vi "ValveFSM.vi"(7 "ReadOnlyIn":T4={"Qref"={"ValveCTR"=refnum, "Error"=refnum}, "UI_EN"=FALSE, "UserEventREF"={"TimeBasedProducer"={"Reg"=refnum, "Ref"=refnum}, "TimeBasedTempRead"={"Reg"=refnum, "Ref"=refnum}}, "UI_REF"=variant, "Paths"={"Log_Dir"=path "", "TempLog"=path "", "WateringLog"=path "", "Error"=path "", "Settings_Dir"=path "", "CFG.ini"=path "", "Plant_Digital_OP"=path "", "TimeTable"=path "", "Consol_Dir"=path "", "Input"=path "", "Output"=path "", "Timeout"=path "", "TimeoutTable"=path "", "Ch_Stat"=path "", "Temp"=path ""}, "PI_REF"={"IO"=enum."Remote", "Interface"=enum."Serial", "LINX Device Config"={"Interface"=enum."Serial", "COM Port"="", "TCP Configuration"={"IP Address"="", "Port"=0}, "Device Family"=0, "Device ID"=0, "Device Name"="", "TCP Ref"=refnum, "Channels"={"DI"=[], "DO"=[], "AI"=[], "AO"=[], "PWM"=[], "QE"=[], "UART"=[], "I2C 2"=[], "SPI"=[], "CAN"=[], "Servo"=[], "AI Ref (V)"=0.0, "AI Resolution (Bits)"=0, "AO Ref (V)"=0.0, "AO Resolution (Bits)"=0}}}, "CFG"={"ProducerEn_PC"=FALSE, "Producer_PC_ms"=0, "ProducerEn_PI"=FALSE, "Producer_PI_ms"=0, "TempLogInterval"=15, "SystemResetTime"=0.0}} {"CFG"."SystemResetTime" format="%<%H:%M:%S>t"}, 8 "error in":errorcluster, 11 "Read_Write_Valv_IN":T1 {"ValidCh" items=["7"=7, "11"=11, "12"=12, "13"=13, "15"=15, "16"=16, "18"=18, "29"=29, "32"=32, "33"=33, "35"=35, "36"=36, "37"=37, "38"=38, "40"=40]}) -> (0 "error out":errorcluster, 3 "Read_Write_Valv_OUT":T1 {"ValidCh" items=["7"=7, "11"=11, "12"=12, "13"=13, "15"=15, "16"=16, "18"=18, "29"=29, "32"=32, "33"=33, "35"=35, "36"=36, "37"=37, "38"=38, "40"=40]}, 4 "Stop":bool)   [LabVIEW 2014, in "ValveCTRL.lvlib"]
uses:
  ValveCTRL.lvlib
  Main/TypeDef/ReadOnly.ctl
  TypeDef/Queue_Cluster.ctl
  TypeDef/States_Enum.ctl
  TypeDef/CHs_List.ctl
  Main/TypeDef/EventData.ctl
  <vilib>/MakerHub/LINX/Private/Type Defs/LINX Ref.ctl
  <vilib>/MakerHub/LINX/Private/Type Defs/Platform.ctl
  <vilib>/MakerHub/LINX/Private/Type Defs/Interface.ctl
  <vilib>/MakerHub/LINX/Private/Device/Type Defs/LINX Device Config.ctl
  <vilib>/MakerHub/LINX/Private/Device/Type Defs/TCP Config.ctl
  <vilib>/MakerHub/LINX/Private/Device/Type Defs/Channels.ctl
  Main/Init/ReadInitCFG/TypeDef/CFG_Cluster.ctl
  TypeDef/Read_Write.ctl
  TypeDef/ChannelStatus.ctl
  Main/Main.lvlib
  TimeBasedProd/TimeBasedProd.lvlib
  <vilib>/MakerHub/LINX/LMH-LINX.lvlib
  <vilib>/MakerHub/LINX/Private/Device/Device.lvlib
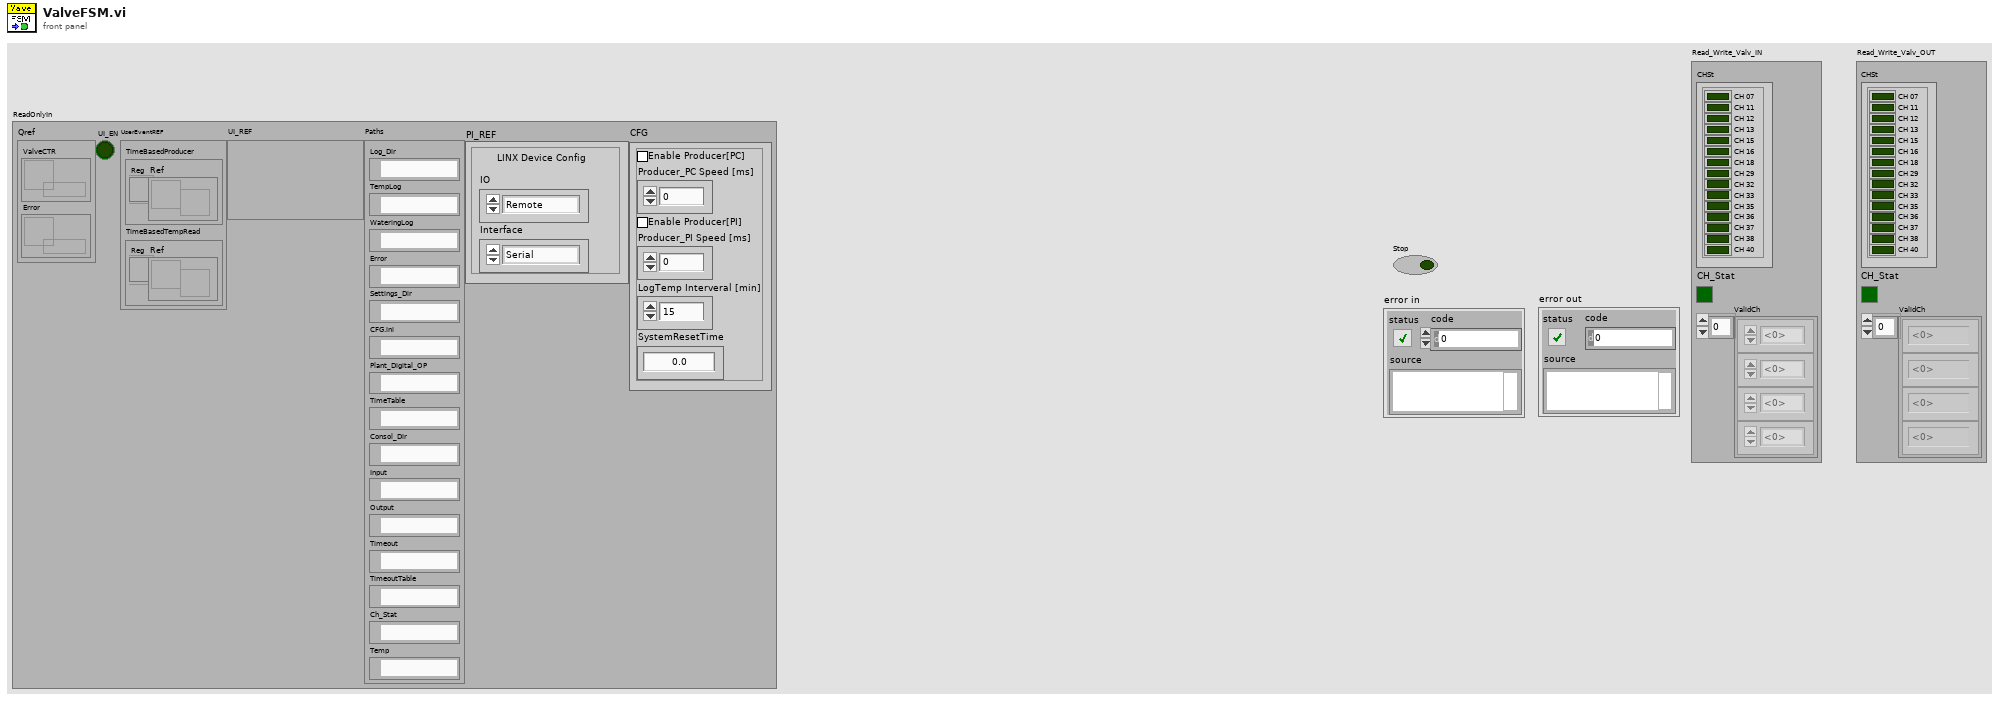
[diagram p1: front panel]
types:
  T1 = typedef "ValveCTRL.lvlib/Read_Write.ctl" = cluster{"CHSt":T2, "CH_Stat":bool, "ValidCh":T3[]}
  T2 = typedef "ValveCTRL.lvlib/ChannelStatus.ctl" = cluster{"CH 07":bool, "CH 11":bool, "CH 12":bool, "CH 13":bool, "CH 15":bool, "CH 16":bool, "CH 18":bool, "CH 29":bool, "CH 32":bool, "CH 33":bool, "CH 35":bool, "CH 36":bool, "CH 37":bool, "CH 38":bool, "CH 40":bool}
  T3 = typedef "ValveCTRL.lvlib/CHs_List.ctl" = u8
  T4 = typedef "Main.lvlib/ReadOnly.ctl" = cluster{"Qref":cluster{"ValveCTR":refnum<queue>, "Error":refnum<queue>}, "UI_EN":bool, "UserEventREF":cluster{"TimeBasedProducer":cluster{"Reg":refnum<event-registration>, "Ref":refnum<user-event>}, "TimeBasedTempRead":cluster{"Reg":refnum<event-registration>, "Ref":refnum<user-event>}}, "UI_REF":variant, "Paths":cluster{"Log_Dir":path, "TempLog":path, "WateringLog":path, "Error":path, "Settings_Dir":path, "CFG.ini":path, "Plant_Digital_OP":path, "TimeTable":path, "Consol_Dir":path, "Input":path, "Output":path, "Timeout":path, "TimeoutTable":path, "Ch_Stat":path, "Temp":path}, "PI_REF":T5, "CFG":T11}
  T5 = typedef "LMH-LINX.lvlib/LINX Ref.ctl" = cluster{"IO":T6, "Interface":T7, "LINX Device Config":T8}
  T6 = typedef "LMH-LINX.lvlib/Platform.ctl" = enum16{"Remote", "Local"}
  T7 = typedef "LMH-LINX.lvlib/Interface.ctl" = enum16{"Serial", "TCP"}
  T8 = typedef "LMH-LINX.lvlib/Device.lvlib/LINX Device Config.ctl" = cluster{"Interface":T7, "COM Port":refnum<visa-resource-name>, "TCP Configuration":T9, "Device Family":u8, "Device ID":u8, "Device Name":string, "TCP Ref":refnum<k5>, "Channels":T10}
  T9 = typedef "LMH-LINX.lvlib/Device.lvlib/TCP Config.ctl" = cluster{"IP Address":string, "Port":u16}
  T10 = typedef "LMH-LINX.lvlib/Channels.ctl" = cluster{"DI":u8[], "DO":u8[], "AI":u8[], "AO":u8[], "PWM":u8[], "QE":u8[], "UART":u8[], "I2C 2":u8[], "SPI":u8[], "CAN":u8[], "Servo":u8[], "AI Ref (V)":dbl, "AI Resolution (Bits)":u8, "AO Ref (V)":dbl, "AO Resolution (Bits)":u8}
  T11 = typedef "Main.lvlib/CFG_Cluster.ctl" = cluster{"ProducerEn_PC":bool, "Producer_PC_ms":u32, "ProducerEn_PI":bool, "Producer_PI_ms":u32, "TempLogInterval":u32, "SystemResetTime":dbl}
  T12 = typedef "ValveCTRL.lvlib/Queue_Cluster.ctl" = cluster{"State":T13, "Channel No":T3, "Duration[S]":dbl}
  T13 = typedef "ValveCTRL.lvlib/States_Enum.ctl" = enum16{"Open Pump", "Open Valve", "Wait Valve", "Close Pump", "Close Valve", "Save State", "StopLoop", "ValidCh"}
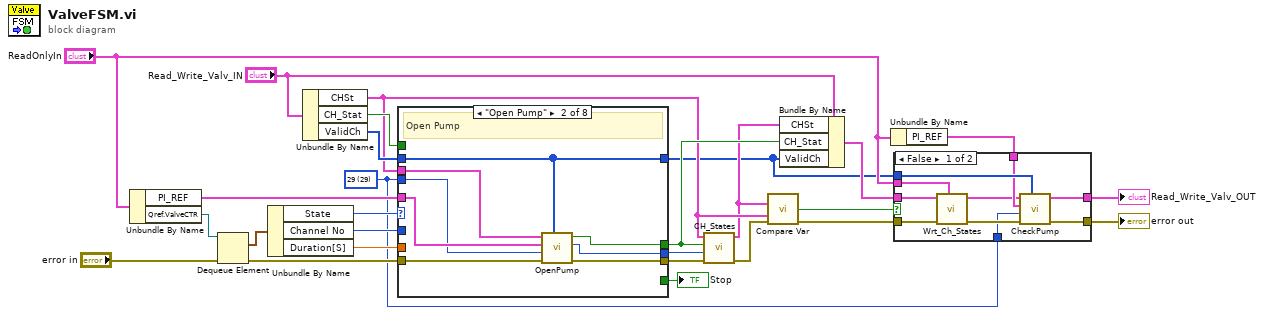
[diagram p0: block diagram]
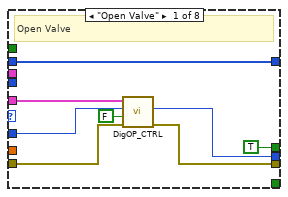
[diagram p3: hidden frame]
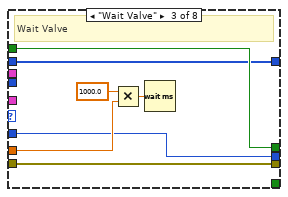
[diagram p4: hidden frame]
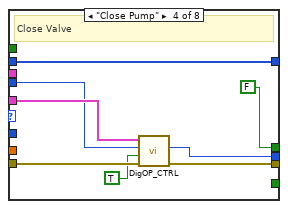
[diagram p5: hidden frame]
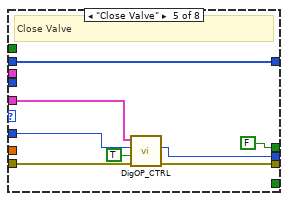
[diagram p6: hidden frame]
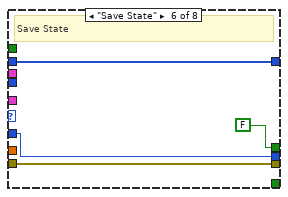
[diagram p7: hidden frame]
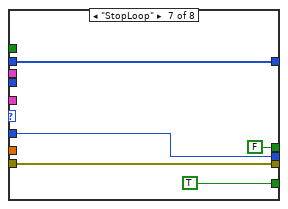
[diagram p8: hidden frame]
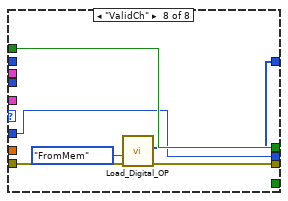
[diagram p9: hidden frame]
diagram:
  w1 = T3 29 items=["7"=7, "11"=11, "12"=12, "13"=13, "15"=15, "16"=16, "18"=18, "29"=29, "32"=32, "33"=33, "35"=35, "36"=36, "37"=37, "38"=38, "40"=40] ("Channel No")
  n1 = Unbundle By Name("ReadOnlyIn") -> ("PI_REF"=w21:T5, "Qref.ValveCTR"=w20:refnum<queue>)
  n2 = Dequeue Element(queue=w20, error in (no error)="error in") -> (element=w22:T12, error out=w26:errorcluster)  [unwired: 1 in, 2 out]
  n3 = Unbundle By Name(w22) -> ("State"=w23:T13, "Channel No"=w24:T3, "Duration[S]"=w25:dbl)
  n4 = Unbundle By Name("Read_Write_Valv_IN") -> ("CHSt"=w13:T2, "CH_Stat"=w16:bool, "ValidCh"=w15:T3[])
  n5 = case shown="\"Open Pump\"" w23 {
    tunnel: w21 -> [w35 w39 _ w58 w66 _ _ _]
    tunnel: w26 -> [w34 w43 w49 w57 w65 w70 w74 w81]
    tunnel: w25 -> [_ _ w50 _ _ _ _ _]
    tunnel: [w33 w42 w49 w55 w63 w70 w74 w80] -> w19
    tunnel: w24 -> [w31 _ w46 _ w62 w68 w73 w78]
    tunnel: [_ _ _ _ _ _ TRUE _] -> w27
    tunnel: w1 -> [_ w38 _ w54 _ _ _ _]
    tunnel: [w30 w41 w46 w53 w61 w68 w73 w78] -> w4
    tunnel: [TRUE w40 w45 FALSE ("Output Value") FALSE ("Output Value") FALSE ("Output Value") FALSE ("Output Value") w79] -> w17
    tunnel: w16 -> [_ _ w45 _ _ _ _ w79]
    tunnel: [w28 w37 w44 w51 w59 w67 w71 w76] -> w3
    tunnel: w15 -> [w28 w37 w44 w51 w59 w67 w71 _]
    tunnel: w13 -> [_ w36 _ _ _ _ _ _]
    frame "Open Valve" {
      # "Open Valve"
      n6 = call "DigOP_CTRL.vi"("Error In"=w34, "Output Value"=FALSE, "Channel No"=w31, "LINX Resource In"=w35) -> ("Error Out"=w33:errorcluster, "Channel No"=w30:T3)  [unwired: 5 in, 1 out]
    }
    frame "Open Pump" {
      # "Open Pump"
      n7 = call "OpenPump.vi"("ValidCh"=w37, "error in"=w43, "Channel No in"=w38, "PI_REF"=w39, "CHStIn"=w36) -> ("error out"=w42:errorcluster, "Channel No out"=w41:T3, "Output Value"=w40:bool)  [unwired: 4 in]
    }
    frame "Wait Valve" {
      # "Wait Valve"
      n8 = Multiply(x=1000.0, y=w50) -> (x*y=w48:dbl)
      n9 = Wait (ms)(milliseconds to wait=w48) -> ()  [unwired: 1 out]
    }
    frame "Close Pump" {
      # "Close Valve"
      n10 = call "DigOP_CTRL.vi"("Error In"=w57, "Output Value"=TRUE, "Channel No"=w54, "LINX Resource In"=w58) -> ("Error Out"=w55:errorcluster, "Channel No"=w53:T3)  [unwired: 5 in, 1 out]
    }
    frame "Close Valve" {
      # "Close Valve"
      n11 = call "DigOP_CTRL.vi"("Error In"=w65, "Output Value"=TRUE, "Channel No"=w62, "LINX Resource In"=w66) -> ("Error Out"=w63:errorcluster, "Channel No"=w61:T3)  [unwired: 5 in, 1 out]
    }
    frame "Save State" {
      # "Save State"
    }
    frame "StopLoop" {
    }
    frame "ValidCh" {
      n12 = call "Load_Digital_OP.vi"("Error In"=w81, "Oper"=enum16{"FromFile", "FromMem"}."FromMem") -> ("Error Out"=w80:errorcluster, "ValidCh"=w76:T3[])  [unwired: 7 in, 1 out]
    }
  }
  "Stop" <- w27
  n13 = call "CH_States.vi"("Error In"=w19, "Channel No"=w4, "State"=w17, "CHStIn"=w13) -> ("Error Out"=w12:errorcluster, "CHStOut"=w6:T2)  [unwired: 6 in]
  n14 = call "Compare Var.vi"("Value 1"=w6, "Value 2"=w13, "error in"=w12) -> ("Equal?"=w11:bool, "error out"=w8:errorcluster)  [unwired: 11 in]
  n15 = Bundle By Name(cluster="Read_Write_Valv_IN", "CHSt"=w6, "CH_Stat"=w17, "ValidCh"=w3) -> (w10:T1)
  n16 = Unbundle By Name("ReadOnlyIn") -> ("PI_REF"=w2:T5)
  n17 = case shown="False" w11 {
    tunnel: w8 -> [w91 w93]
    tunnel: w10 -> [w90 w92]
    tunnel: [w82 w92] -> w9
    tunnel: [w87 w93] -> w5
    tunnel: "ReadOnlyIn" -> [w89 _]
    tunnel: w1 -> [w86 _]
    tunnel: w3 -> [w85 _]
    tunnel: w2 -> [w84 _]
    frame False {
      n18 = call "Wrt_Ch_States.vi"("ReadOnlyIn"=w89, "error in (no error)"=w91, "Read_Write_Valv_IN"=w90) -> ("error out"=w88:errorcluster, "Read_Write_Valv_OUT"=w83:T1)  [unwired: 7 in]
      n19 = call "CheckPump.vi"("ValidCh"=w85, "error in"=w88, "Channel No in"=w86, "PI_REF"=w84, "Read_Write_Valv_IN"=w83) -> ("error out"=w87:errorcluster, "Read_Write_Valv_OUT"=w82:T1)  [unwired: 5 in]
    }
    frame True {
    }
  }
  "error out" <- w5
  "Read_Write_Valv_OUT" <- w9
